vi "Configure Device.vi"(8 "error in (no error)":errorcluster, 10 "Max Beams":dbl, 11 "Toggle 6 in":refnum<class "Toggle 6.lvclass">) -> (0 "error out":errorcluster, 3 "Toggle 6 out":refnum<class "Toggle 6.lvclass">)   [LabVIEW 2020, in "Toggle 6.lvclass"]
doc: "Interface for configuring the device for testing"
uses:
  Toggle 6.lvclass
  C:/Sandbox/Git_Sandbox/WiSpry Test Framework source code (LV20)/WiSpry Test Framework/Devices/Device.lvclass
  Controls/EFuse modes enum.ctl
  Controls/Configure decive refs cluster.ctl
  Controls/Parameter Cluster.ctl
  Controls/DC Offset Cluster.ctl
  Instruments/Power Supply/Power Supply.lvclass
  Device.lvclass
panel:
  in  "Enable DC Offset":bool
  in  "DC Offset":enum32{"From To", "Array"}(tab)
  in  "From To Cluster DC Offset":cluster{"From":dbl, "To":dbl, "Step":dbl} {"Step" min=0.0; "From" min=0.0}
  in  "Array DC Offset":dbl[](array[numeric]) min=0.0
  in  "Efuse Multiplier":T1
  in  "Enable Charge Pump":bool
  in  "Charge Pump":enum32{"From To", "Array"}(tab)
  in  "From To Cluster Charge Pump":cluster{"From":dbl, "To":dbl, "Step":dbl}={"From"=29.75, "To"=29.75, "Step"=0.75} {"Step" min=0.75 max=50.0 step=0.75; "To" min=29.75 max=50.0 step=0.75; "From" min=29.75 max=50.0 step=0.75}
  in  "Array Charge Pump":dbl[](array[numeric]) min=29.75 max=50.0 step=0.75
  in  "OK Button":bool
  in  "Enable Register 4":bool
  in  "Register 4":enum32{"From To", "Array"}(tab)
  in  "From To Cluster Register 4":cluster{"From":dbl, "To":dbl, "Step":dbl} {"Step" min=0.125 max=1.875 step=0.125; "To" min=0.0 max=1.875 step=0.125; "From" min=0.0 max=1.875 step=0.125}
  in  "Array Register 4":dbl[](array[numeric]) min=0.0 max=1.875 step=0.125
  in  "Enable Register 3":bool
  in  "Register 3":enum32{"From To", "Array"}(tab)
  in  "From To Cluster Register 3":cluster{"From":dbl, "To":dbl, "Step":dbl} {"Step" min=0.0625 max=1.8125 step=0.0625; "To" min=0.0 max=1.8125 step=0.0625; "From" min=0.0 max=1.8125 step=0.0625}
  in  "Array Register 3":dbl[](array[numeric]) min=0.0 max=1.8125 step=0.0625
  in  "Enable Register 2":bool
  in  "Register 2":enum32{"From To", "Array"}(tab)
  in  "From To Cluster Register 2":cluster{"From":dbl, "To":dbl, "Step":dbl} {"Step" min=0.0625 max=1.8125 step=0.0625; "To" min=0.0 max=1.8125 step=0.0625; "From" min=0.0 max=1.8125 step=0.0625}
  in  "Array Register 2":dbl[](array[numeric]) min=0.0 max=1.8125 step=0.0625
  in  "Enable Register 1":bool
  in  "Register 1":enum32{"From To", "Array"}(tab)
  in  "From To Cluster Register 1":cluster{"From":dbl, "To":dbl, "Step":dbl} {"Step" min=0.125 max=1.875 step=0.125; "To" min=0.0 max=1.875 step=0.125; "From" min=0.0 max=1.875 step=0.125}
  in  "Array Register 1":dbl[](array[numeric]) min=0.0 max=1.875 step=0.125
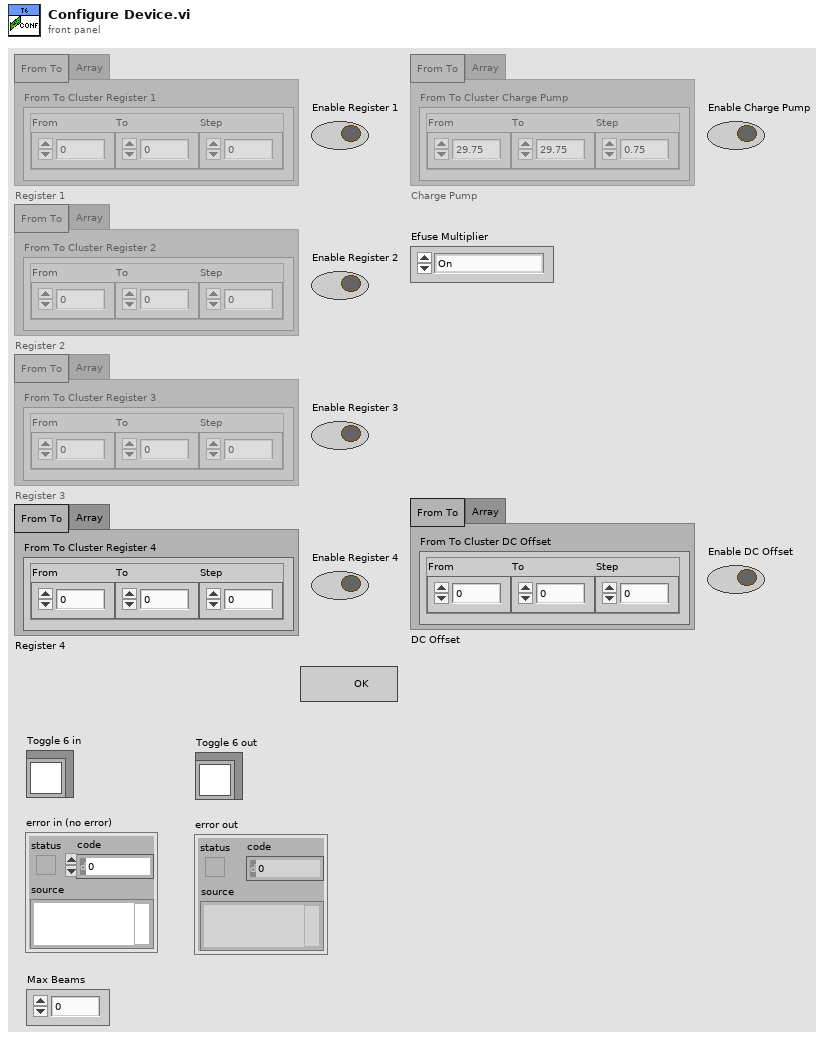
[diagram p1: front panel]
types:
  T1 = typedef "Toggle 6.lvclass/EFuse modes enum.ctl" = enum16{"On", "Off", "Both On and Off"}
  T2 = typedef "Toggle 6.lvclass/Configure decive refs cluster.ctl" = cluster{"Enable Register 1":refnum<vi>, "Register 1":refnum<vi>, "Array Register 1":refnum<vi>, "From To Cluster Register 1":refnum<vi>, "Enable Register 2":refnum<vi>, "Register 2":refnum<vi>, "Array Register 2":refnum<vi>, "From To Cluster Register 2":refnum<vi>, "Enable Register 3":refnum<vi>, "Register 3":refnum<vi>, "Array Register 3":refnum<vi>, "From To Cluster Register 3":refnum<vi>, "Enable Register 4":refnum<vi>, "Register 4":refnum<vi>, "Array Register 4":refnum<vi>, "From To Cluster Register 4":refnum<vi>, "Enable Charge Pump":refnum<vi>, "Charge Pump":refnum<vi>, "Array Charge Pump":refnum<vi>, "From To Cluster Charge Pump":refnum<vi>, "Efuse Multiplier":refnum<vi>, "Enable DC Offset":refnum<vi>, "DC Offset":refnum<vi>, "Array DC Offset":refnum<vi>, "From To Cluster DC Offset":refnum<vi>}
  T3 = typedef "Device.lvclass/DC Offset Cluster.ctl" = cluster{"Enable":bool, "Use Array":bool, "Array":dbl[], "To From Cluster":cluster{"From":dbl, "To":dbl, "Step":dbl}, "Current Value":dbl, "DC Offset":refnum<class "Power Supply.lvclass">}
  T4 = typedef "Toggle 6.lvclass/Parameter Cluster.ctl" = cluster{"Enable":bool, "Register Number":u32, "Use Array":bool, "Array":dbl[], "To From Cluster":cluster{"From":dbl, "To":dbl, "Step":dbl}}
  T5 = enum8{"Enabled", "Disabled", "Disabled and Grayed Out"}
  T6 = typedef "Device.lvclass/Device Information Cluster.ctl" = cluster{"Device Info":string[][], "Default Values":T7[], "Fetched info":string[][]}
  T7 = typedef "PIC-Device.lvclass/Register to Write.ctl" = cluster{"Register":u32, "Value":u32, "Dev Address":u32, "Physical Adress":u32}
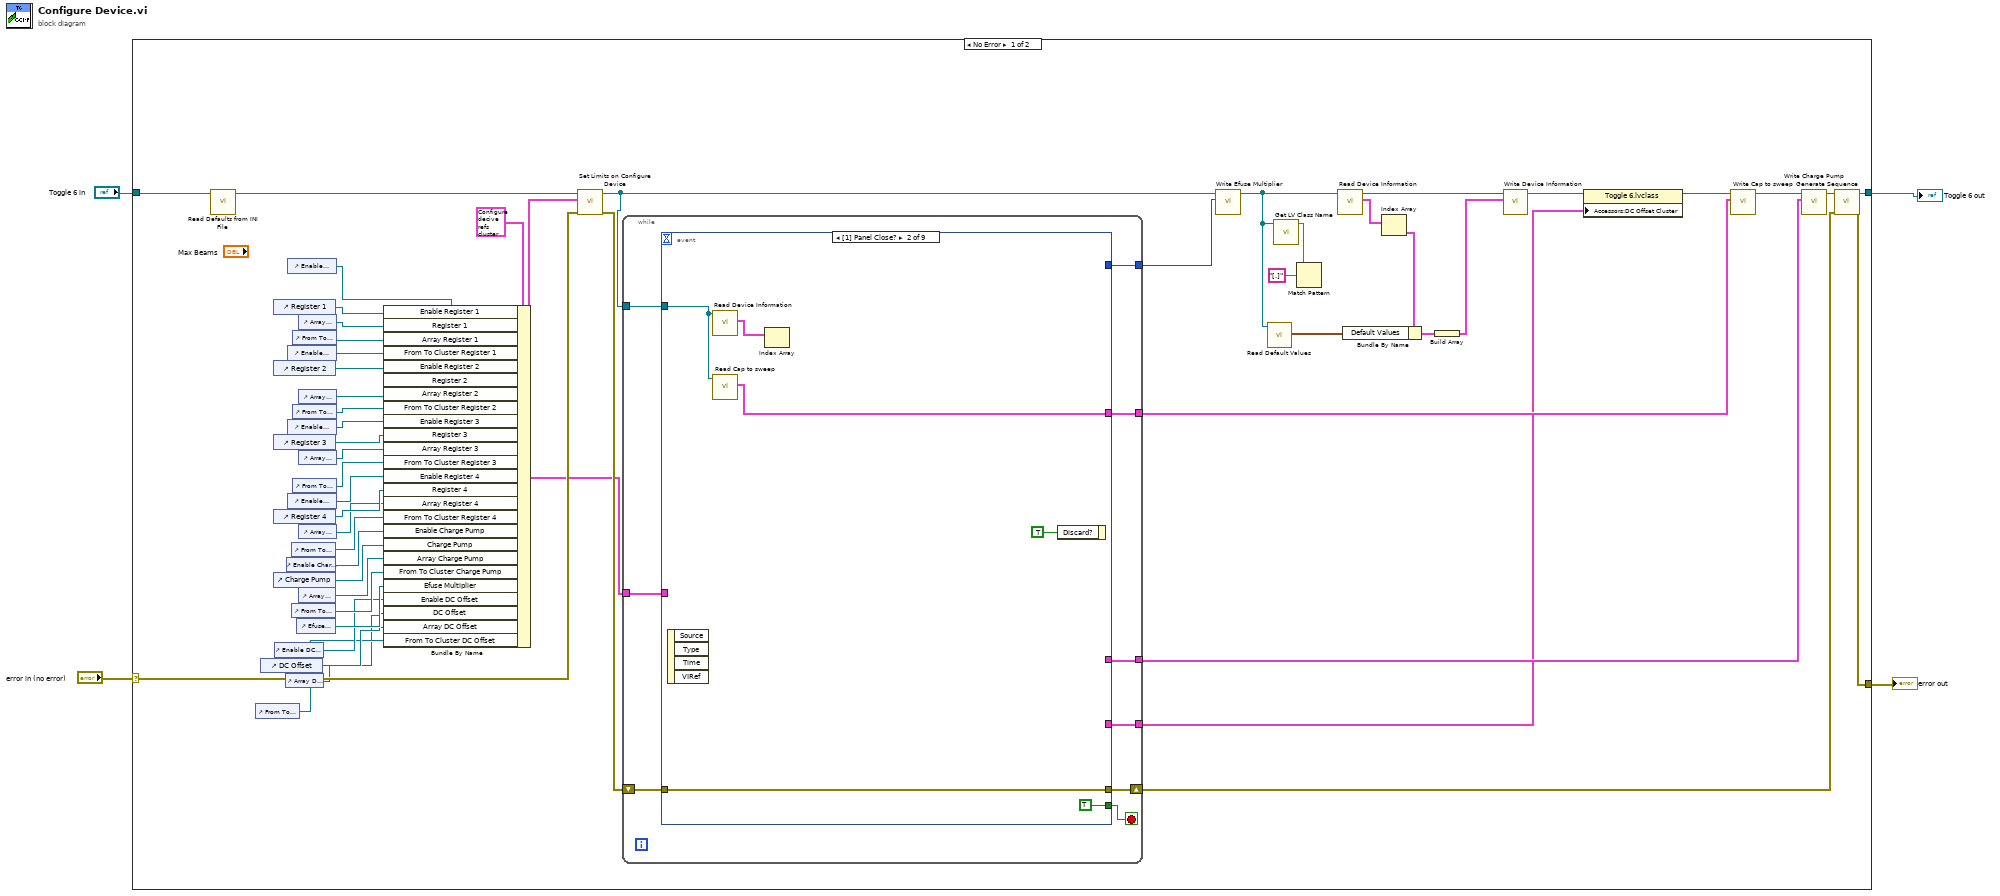
[diagram p0: block diagram]
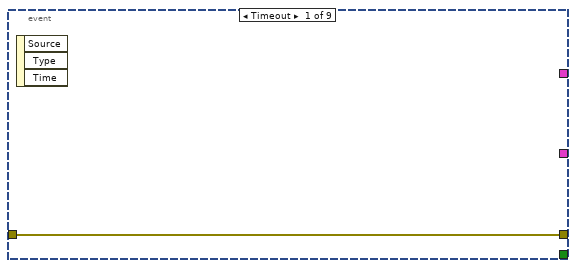
[diagram p2: hidden frame]
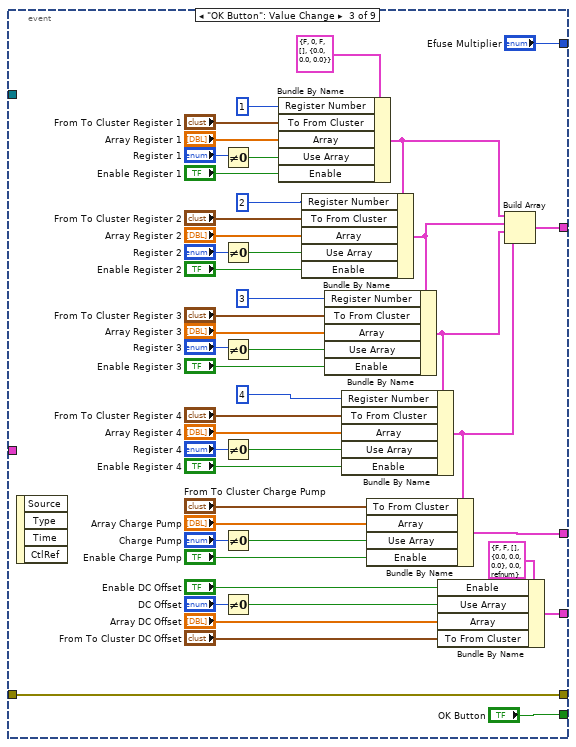
[diagram p3: hidden frame]
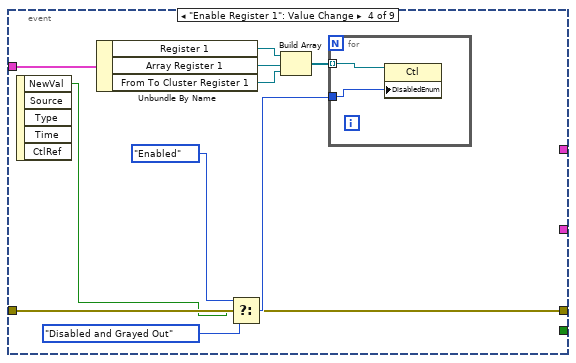
[diagram p4: hidden frame]
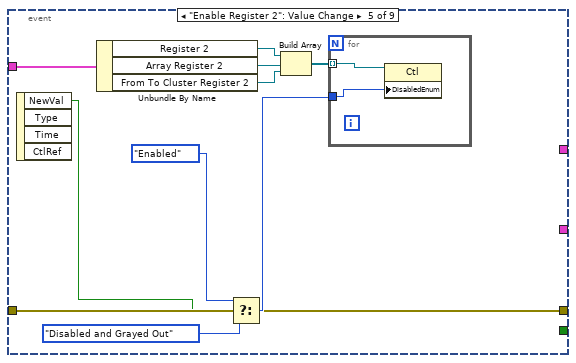
[diagram p5: hidden frame]
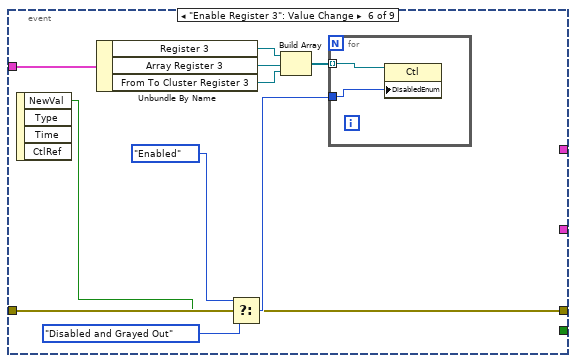
[diagram p6: hidden frame]
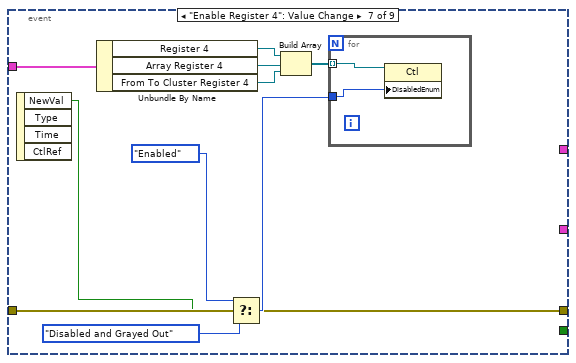
[diagram p7: hidden frame]
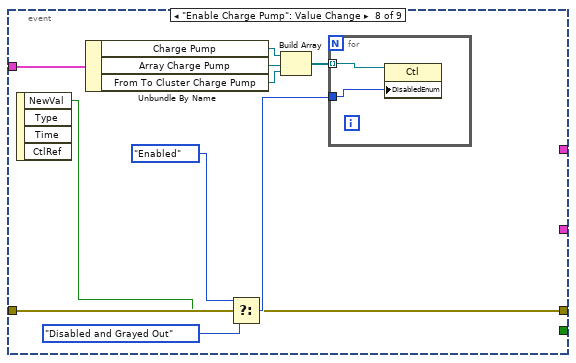
[diagram p8: hidden frame]
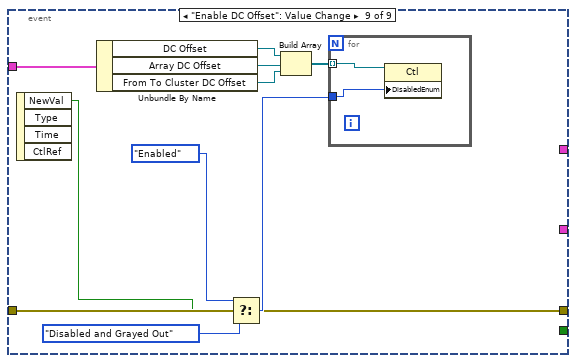
[diagram p9: hidden frame]
diagram:
  n1 = case shown="No Error" "error in (no error)" {
    selector: "error in (no error)" -> [w33 w192]
    tunnel: "Toggle 6 in" -> [w28 w191]
    tunnel: [w23 w192] -> w2
    tunnel: [w25 w191] -> w1
    frame No Error {
      n2 = call "Read Defaults from INI File.vi"("Toggle 6 in"=w28) -> ("Toggle 6 out"=w27:refnum<class "Toggle 6.lvclass">)  [unwired: 9 in, 1 out]
      n3 = control-ref of="From To Cluster DC Offset"() -> (w14:refnum<vi>)
      n4 = control-ref of="DC Offset"() -> (w12:refnum<vi>)
      n5 = control-ref of="Charge Pump"() -> (w37:refnum<vi>)
      n6 = control-ref of="Register 1"() -> (w53:refnum<vi>)
      n7 = control-ref of="Register 2"() -> (w49:refnum<vi>)
      n8 = control-ref of="Register 3"() -> (w45:refnum<vi>)
      n9 = control-ref of="Register 4"() -> (w41:refnum<vi>)
      n10 = control-ref of="Enable DC Offset"() -> (w16:refnum<vi>)
      n11 = control-ref of="Array DC Offset"() -> (w15:refnum<vi>)
      n12 = control-ref of="Enable Charge Pump"() -> (w38:refnum<vi>)
      n13 = control-ref of="Enable Register 1"() -> (w54:refnum<vi>)
      n14 = control-ref of="Enable Register 2"() -> (w50:refnum<vi>)
      n15 = control-ref of="Enable Register 3"() -> (w46:refnum<vi>)
      n16 = control-ref of="Enable Register 4"() -> (w42:refnum<vi>)
      n17 = control-ref of="From To Cluster Register 4"() -> (w39:refnum<vi>)
      n18 = control-ref of="From To Cluster Charge Pump"() -> (w35:refnum<vi>)
      n19 = control-ref of="From To Cluster Register 1"() -> (w51:refnum<vi>)
      n20 = control-ref of="From To Cluster Register 2"() -> (w47:refnum<vi>)
      n21 = control-ref of="From To Cluster Register 3"() -> (w43:refnum<vi>)
      n22 = control-ref of="Efuse Multiplier"() -> (w34:refnum<vi>)
      n23 = control-ref of="Array Charge Pump"() -> (w36:refnum<vi>)
      n24 = control-ref of="Array Register 1"() -> (w52:refnum<vi>)
      n25 = control-ref of="Array Register 2"() -> (w48:refnum<vi>)
      n26 = control-ref of="Array Register 3"() -> (w44:refnum<vi>)
      n27 = control-ref of="Array Register 4"() -> (w40:refnum<vi>)
      n28 = Bundle By Name(cluster=T2 {"Enable Register 1"=refnum, "Register 1"=refnum, "Array Register 1"=refnum, "From To Cluster Register 1"=refnum, "Enable Register 2"=refnum, "Register 2"=refnum, "Array Register 2"=refnum, "From To Cluster Register 2"=refnum, "Enable Register 3"=refnum, "Register 3"=refnum, "Array Register 3"=refnum, "From To Cluster Register 3"=refnum, "Enable Register 4"=refnum, "Register 4"=refnum, "Array Register 4"=refnum, "From To Cluster Register 4"=refnum, "Enable Charge Pump"=refnum, "Charge Pump"=refnum, "Array Charge Pump"=refnum, "From To Cluster Charge Pump"=refnum, "Efuse Multiplier"=refnum, "Enable DC Offset"=refnum, "DC Offset"=refnum, "Array DC Offset"=refnum, "From To Cluster DC Offset"=refnum}, "Enable Register 1"=w54, "Register 1"=w53, "Array Register 1"=w52, "From To Cluster Register 1"=w51, "Enable Register 2"=w50, "Register 2"=w49, "Array Register 2"=w48, "From To Cluster Register 2"=w47, "Enable Register 3"=w46, "Register 3"=w45, "Array Register 3"=w44, "From To Cluster Register 3"=w43, "Enable Register 4"=w42, "Register 4"=w41, "Array Register 4"=w40, "From To Cluster Register 4"=w39, "Enable Charge Pump"=w38, "Charge Pump"=w37, "Array Charge Pump"=w36, "From To Cluster Charge Pump"=w35, "Efuse Multiplier"=w34, "Enable DC Offset"=w16, "DC Offset"=w12, "Array DC Offset"=w15, "From To Cluster DC Offset"=w14) -> (w31:T2)
      n29 = call "Set Limits on Configure Device.vi"("error in (no error)"=w33, "cluster"=w31, "Toggle 6 in"=w27) -> ("error out"=w32:errorcluster, "Toggle 6 out"=w13:refnum<class "Toggle 6.lvclass">)  [unwired: 7 in]
      n30 = while {
        shift-right: [w63] -> w24
        shift-left: w32 -> [w62]
        tunnel: w31 -> [w64]
        tunnel: [w61] -> w55
        tunnel: [w60] -> w29
        tunnel: [w59] -> w22
        tunnel: w13 -> [w58]
        tunnel: [w57] -> w5
        stop <- w65 stop-if-true
        n31 = event shown="[1] Panel Close?" {
          selector: _ -> [_ _ _ _ _ _ _ _ _]
          dyn-events: _ -> [_ _ _ _ _ _ _ _ _]
          timeout: _ -> [_ _ _ _ _ _ _ _ _]
          tunnel: [_ TRUE ("OK Button") "OK Button" _ _ _ _ _ _] -> w65
          tunnel: w64 -> [_ _ _ w128 w140 w152 w164 w176 w188]
          tunnel: [w66 w72 w117 w120 w132 w144 w156 w168 w180] -> w63
          tunnel: w62 -> [w66 w72 w117 w120 w132 w144 w156 w168 w180]
          tunnel: [_ _ w95 _ _ _ _ _ _] -> w61
          tunnel: [_ w69 w85 _ _ _ _ _ _] -> w60
          tunnel: [_ _ "Efuse Multiplier" _ _ _ _ _ _] -> w59
          tunnel: w58 -> [_ w70 _ _ _ _ _ _ _]
          tunnel: [_ _ w74 _ _ _ _ _ _] -> w57
          event Timeout {
            n32 = event-data() -> ()  [unwired: 1 in, 3 out]
          }
          event Panel Close? {
            n33 = event-data() -> ()  [unwired: 1 in, 4 out]
            n34 = call-dynamic "Read Device Information.vi"("Device in"=w70) -> ("Device Info"=w71:T6[])  [unwired: 8 in, 2 out]
            n35 = call-dynamic "Read Cap to sweep.vi"("Toggle 6 in"=w70) -> ("Cap to sweep"=w69:T4[])  [unwired: 9 in, 1 out]
            n36 = Index Array(array=w71) -> ()  [unwired: 1 in, 1 out]
            n37 = event-data("Discard?"=TRUE) -> ()  [unwired: 1 in, 1 out]
          }
          event "OK Button": Value Change {
            n38 = event-data() -> ()  [unwired: 1 in, 4 out]
            n39 = Not Equal To 0?(x="Register 1") -> (x != 0?=w99:bool)
            n40 = Not Equal To 0?(x="Register 2") -> (x != 0?=w104:bool)
            n41 = Not Equal To 0?(x="Register 3") -> (x != 0?=w108:bool)
            n42 = Not Equal To 0?(x="Register 4") -> (x != 0?=w112:bool)
            n43 = Not Equal To 0?(x="Charge Pump") -> (x != 0?=w116:bool)
            n44 = Not Equal To 0?(x="DC Offset") -> (x != 0?=w77:bool)
            n45 = Bundle By Name(cluster=T4 {"Enable"=FALSE, "Register Number"=0, "Use Array"=FALSE, "Array"=[], "To From Cluster"={"From"=0.0, "To"=0.0, "Step"=0.0}} ("output cluster"), "Register Number"=u32 1, "To From Cluster"="From To Cluster Register 1", "Array"="Array Register 1", "Use Array"=w99, "Enable"="Enable Register 1") -> (w89:T4)
            n46 = Bundle By Name(cluster=w89, "Register Number"=u32 2, "To From Cluster"="From To Cluster Register 2", "Array"="Array Register 2", "Use Array"=w104, "Enable"="Enable Register 2") -> (w88:T4)
            n47 = Bundle By Name(cluster=w88, "Register Number"=u32 3, "To From Cluster"="From To Cluster Register 3", "Array"="Array Register 3", "Use Array"=w108, "Enable"="Enable Register 3") -> (w87:T4)
            n48 = Bundle By Name(cluster=w87, "Register Number"=u32 4, "To From Cluster"="From To Cluster Register 4", "Array"="Array Register 4", "Use Array"=w112, "Enable"="Enable Register 4") -> (w86:T4)
            n49 = Bundle By Name(cluster=w86, "To From Cluster"="From To Cluster Charge Pump", "Array"="Array Charge Pump", "Use Array"=w116, "Enable"="Enable Charge Pump") -> (w95:T4)
            n50 = Bundle By Name(cluster=T3 {"Enable"=FALSE, "Use Array"=FALSE, "Array"=[], "To From Cluster"={"From"=0.0, "To"=0.0, "Step"=0.0}, "Current Value"=0.0, "DC Offset"=refnum} ("DC Offset Cluster"), "Enable"="Enable DC Offset", "Use Array"=w77, "Array"="Array DC Offset", "To From Cluster"="From To Cluster DC Offset") -> (w74:T3)
            n51 = Build Array(w89, w88, w87, w86) -> (w85:T4[])
          }
          event "Enable Register 1": Value Change {
            n52 = event-data() -> ("NewVal"=w119:bool)  [unwired: 1 in, 4 out]
            n53 = Unbundle By Name(w128) -> ("Register 1"=w127:refnum<vi>, "Array Register 1"=w126:refnum<vi>, "From To Cluster Register 1"=w125:refnum<vi>)
            n54 = Select(t=T5."Enabled" ("Disabled"), s=w119, f=T5."Disabled and Grayed Out") -> (s? t:f=w123:T5)
            n55 = Build Array(w127, w126, w125) -> (w124:refnum<vi>[])
            n56 = for {
              tunnel: w124 -> [w130] mode=indexing
              tunnel: w123 -> [w129]
              n57 = property class="Ctl"(reference=w130, "DisabledEnum"=w129) -> ()  [unwired: 1 in, 2 out]
            }
          }
          event "Enable Register 2": Value Change {
            n58 = event-data() -> ("NewVal"=w131:bool)  [unwired: 1 in, 3 out]
            n59 = Unbundle By Name(w140) -> ("Register 2"=w139:refnum<vi>, "Array Register 2"=w138:refnum<vi>, "From To Cluster Register 2"=w137:refnum<vi>)
            n60 = Select(t=T5."Enabled" ("Disabled"), s=w131, f=T5."Disabled and Grayed Out") -> (s? t:f=w135:T5)
            n61 = Build Array(w139, w138, w137) -> (w136:refnum<vi>[])
            n62 = for {
              tunnel: w136 -> [w142] mode=indexing
              tunnel: w135 -> [w141]
              n63 = property class="Ctl"(reference=w142, "DisabledEnum"=w141) -> ()  [unwired: 1 in, 2 out]
            }
          }
          event "Enable Register 3": Value Change {
            n64 = event-data() -> ("NewVal"=w143:bool)  [unwired: 1 in, 3 out]
            n65 = Unbundle By Name(w152) -> ("Register 3"=w151:refnum<vi>, "Array Register 3"=w150:refnum<vi>, "From To Cluster Register 3"=w149:refnum<vi>)
            n66 = Select(t=T5."Enabled" ("Disabled"), s=w143, f=T5."Disabled and Grayed Out") -> (s? t:f=w147:T5)
            n67 = Build Array(w151, w150, w149) -> (w148:refnum<vi>[])
            n68 = for {
              tunnel: w148 -> [w154] mode=indexing
              tunnel: w147 -> [w153]
              n69 = property class="Ctl"(reference=w154, "DisabledEnum"=w153) -> ()  [unwired: 1 in, 2 out]
            }
          }
          event "Enable Register 4": Value Change {
            n70 = event-data() -> ("NewVal"=w155:bool)  [unwired: 1 in, 3 out]
            n71 = Unbundle By Name(w164) -> ("Register 4"=w163:refnum<vi>, "Array Register 4"=w162:refnum<vi>, "From To Cluster Register 4"=w161:refnum<vi>)
            n72 = Select(t=T5."Enabled" ("Disabled"), s=w155, f=T5."Disabled and Grayed Out") -> (s? t:f=w159:T5)
            n73 = Build Array(w163, w162, w161) -> (w160:refnum<vi>[])
            n74 = for {
              tunnel: w160 -> [w166] mode=indexing
              tunnel: w159 -> [w165]
              n75 = property class="Ctl"(reference=w166, "DisabledEnum"=w165) -> ()  [unwired: 1 in, 2 out]
            }
          }
          event "Enable Charge Pump": Value Change {
            n76 = event-data() -> ("NewVal"=w167:bool)  [unwired: 1 in, 3 out]
            n77 = Unbundle By Name(w176) -> ("Charge Pump"=w175:refnum<vi>, "Array Charge Pump"=w174:refnum<vi>, "From To Cluster Charge Pump"=w173:refnum<vi>)
            n78 = Select(t=T5."Enabled" ("Disabled"), s=w167, f=T5."Disabled and Grayed Out") -> (s? t:f=w171:T5)
            n79 = Build Array(w175, w174, w173) -> (w172:refnum<vi>[])
            n80 = for {
              tunnel: w172 -> [w178] mode=indexing
              tunnel: w171 -> [w177]
              n81 = property class="Ctl"(reference=w178, "DisabledEnum"=w177) -> ()  [unwired: 1 in, 2 out]
            }
          }
          event "Enable DC Offset": Value Change {
            n82 = event-data() -> ("NewVal"=w179:bool)  [unwired: 1 in, 3 out]
            n83 = Unbundle By Name(w188) -> ("DC Offset"=w187:refnum<vi>, "Array DC Offset"=w186:refnum<vi>, "From To Cluster DC Offset"=w185:refnum<vi>)
            n84 = Select(t=T5."Enabled" ("Disabled"), s=w179, f=T5."Disabled and Grayed Out") -> (s? t:f=w183:T5)
            n85 = Build Array(w187, w186, w185) -> (w184:refnum<vi>[])
            n86 = for {
              tunnel: w184 -> [w190] mode=indexing
              tunnel: w183 -> [w189]
              n87 = property class="Ctl"(reference=w190, "DisabledEnum"=w189) -> ()  [unwired: 1 in, 2 out]
            }
          }
        }
      }
      n88 = call-dynamic "Write Efuse Multiplier.vi"("Efuse Multiplier"=w22, "Toggle 6 in"=w13) -> ("Toggle 6 out"=w11:refnum<class "Toggle 6.lvclass">)  [unwired: 9 in]
      n89 = call-dynamic "Read Default Values.vi"("Toggle 6 in"=w11) -> ("Default Values"=w20:T7[])  [unwired: 9 in, 1 out]
      n90 = call <vilib>:"Get LV Class Name.vi"("object"=w11) -> ("class name"=w21:string)  [unwired: 9 in, 1 out]
      n91 = Match Pattern(string=w21, regular expression="[.]") -> ()  [unwired: 1 in, 4 out]
      n92 = call-dynamic "Read Device Information.vi"("Device in"=w11) -> ("Device Info"=w9:T6[], "Device out"=w10:refnum<class "Toggle 6.lvclass">)  [unwired: 8 in, 1 out]
      n93 = Index Array(array=w9) -> (element=w8:T6)  [unwired: 1 in]
      n94 = Bundle By Name(cluster=w8, "Default Values"=w20) -> (w19:T6)
      n95 = Build Array(w19) -> (w18:T6[])
      n96 = call-dynamic "Write Device Information.vi"("Device Info"=w18, "Device in"=w10) -> ("Device out"=w7:refnum<class "Toggle 6.lvclass">)  [unwired: 8 in, 1 out]
      n97 = property class="Toggle 6.lvclass"(reference=w7, "Accessors:DC Offset Cluster"=w5) -> (reference out=w6:refnum<class "Toggle 6.lvclass">)  [unwired: 1 in, 1 out]
      n98 = call-dynamic "Write Cap to sweep.vi"("Cap to sweep"=w29, "Toggle 6 in"=w6) -> ("Toggle 6 out"=w30:refnum<class "Toggle 6.lvclass">)  [unwired: 9 in]
      n99 = call-dynamic "Write Charge Pump.vi"("Parameter Cluster"=w55, "Toggle 6 in"=w30) -> ("Toggle 6 out"=w26:refnum<class "Toggle 6.lvclass">)  [unwired: 8 in, 1 out]
      n100 = call "Generate Sequence.vi"("error in (no error)"=w24, "Toggle 6 in"=w26) -> ("error out"=w23:errorcluster, "Toggle 6 out"=w25:refnum<class "Toggle 6.lvclass">)  [unwired: 8 in]
    }
    frame Error {
    }
  }
  "error out" <- w2
  "Toggle 6 out" <- w1
